vi "Folder to first and last B Field.vi"(9 "B Field":i32, 10 "Wavenames":string[](array[string]), 11 "path":path) -> (2 "B Start":dbl, 3 "B Latest":dbl)   [LabVIEW 2016]
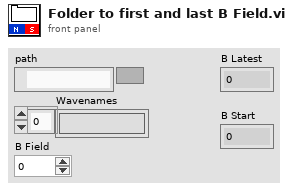
[diagram p1: front panel]
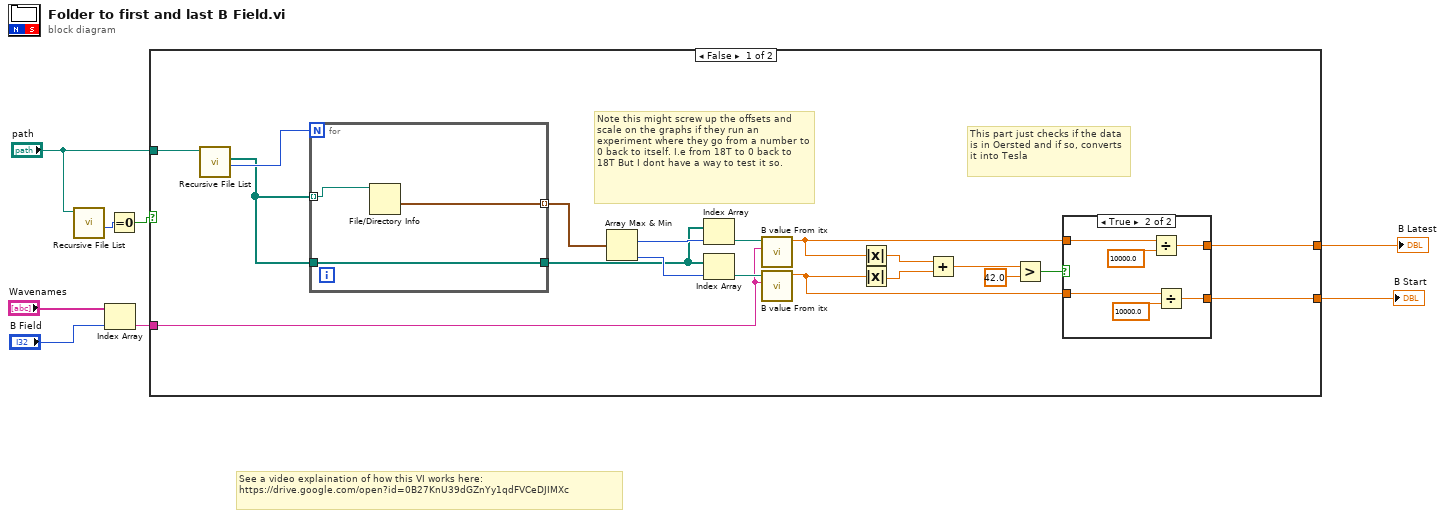
[diagram p0: block diagram]
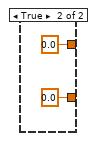
[diagram p3: hidden frame]
diagram:
  # "See a video explaination of how this VI works here: \nhttps://drive.google.com/open?id=0B27KnU39dGZnYy1qdFVCeDJIMXc"
  n1 = call <vilib>:"Recursive File List.vi"("Folder Path"="path") -> ("Number of Files"=w5:i32)  [unwired: 6 in, 4 out]
  n2 = Index Array(array="Wavenames", index="B Field") -> (element=w1:string)
  n3 = Equal To 0?(x=w5) -> (x = 0?=w4:bool)
  n4 = case shown="False" w4 {
    tunnel: "path" -> [w21 _]
    tunnel: [w18 0.0 ("Numeric")] -> w8
    tunnel: [w17 0.0 ("Numeric")] -> w7
    tunnel: w1 -> [w9 _]
    frame False {
      # "This part just checks if the data is in Oersted and if so, converts it into Tesla"
      # "Note this might screw up the offsets and scale on the graphs if they run an experiment where they go from a number to 0 back to itself. I.e from 18T to 0 back to 18T But I dont have a way to test it so."
      n5 = call <vilib>:"Recursive File List.vi"("Folder Path"=w21) -> ("Number of Files"=w27:i32, "All Files in Dir"=w19:path[])  [unwired: 6 in, 3 out]
      n6 = for {
        N: w27 -> [_]
        tunnel: w19 -> [w37] mode=indexing
        tunnel: [w36] -> w22 mode=indexing
        tunnel: [w38] -> w20
        tunnel: w19 -> [w38]
        n7 = File/Directory Info(path=w37) -> (last mod=w36:timestamp)  [unwired: 1 in, 6 out]
      }
      n8 = Array Max & Min(array=w22) -> (max index (indices)=w23:i32, min index (indices)=w26:i32)  [unwired: 2 out]
      n9 = Index Array(array=w20, index=w23) -> (element=w25:path)
      n10 = Index Array(array=w20, index=w26) -> (element=w24:path)
      n11 = call "B value From itx.vi"("B Field Name"=w9, "file (use dialog)"=w25) -> ("Numeric"=w11:dbl)  [unwired: 9 in]
      n12 = call "B value From itx.vi"("B Field Name"=w9, "file (use dialog)"=w24) -> ("Numeric"=w10:dbl)  [unwired: 9 in]
      n13 = Absolute Value(x=w11) -> (abs(x)=w16:dbl)
      n14 = Absolute Value(x=w10) -> (abs(x)=w15:dbl)
      n15 = Add(x=w16, y=w15) -> (x+y=w14:dbl)
      n16 = Greater?(x=w14, y=42.0) -> (0:w12:bool)
      n17 = case shown="True" w12 {
        tunnel: w10 -> [w28 w35]
        tunnel: [w29 w34] -> w18
        tunnel: [w28 w33] -> w17
        tunnel: w11 -> [w29 w30]
        frame False {
        }
        frame True {
          n18 = Divide(x=w30, y=10000.0) -> (x/y=w34:dbl)
          n19 = Divide(x=w35, y=10000.0) -> (x/y=w33:dbl)
        }
      }
    }
    frame True {
    }
  }
  "B Latest" <- w8
  "B Start" <- w7
